vi "play_nPoint_id_slew_OL_FIFO.vi"() -> ()   [LabVIEW 2017]
uses:
  <vilib>/userdefined/High Color/nirio_resource_hc.ctl
  <vilib>/Utility/file.llb/Read Delimited Spreadsheet (DBL).vi
  <vilib>/FPGAPlugInAG/cRIO-9082/niLvFpga_Open_cRIO-9082.vi
  <vilib>/rvi/interface/common/dynamic/niFpgaDynamicAddResources.vi
  <vilib>/FPGAPlugInAG/Dynamic/niLvFpga_Reset_Dynamic.vi
  <vilib>/rvi/interface/common/niFpgaWaitOnOcc.vi
  <vilib>/Utility/error.llb/Error Cluster From Error Code.vi
  <vilib>/rvi/errors/niLvFpgaAdjustHostInterfaceError.vi
  <vilib>/FPGAPlugInAG/Dynamic/niLvFpga_Run_Dynamic.vi
  <vilib>/Utility/file.llb/Write Delimited Spreadsheet (DBL).vi
  <vilib>/FPGAPlugInAG/Dynamic/niLvFpga_Close_Dynamic.vi
  <vilib>/rvi/interface/nirviOpenFPGA/nirviOpenFPGA.xnode
  FPGA Bitfiles/XYpeizocontrol_FPGATargetSPARTA_nPointidslewOLFI_Q7UGYaeAAEs.lvbitx
  <vilib>/rvi/interface/nirviMethod/nirviMethod.xnode
  <vilib>/rvi/interface/nirviReadWriteControl/nirviReadWriteControl.xnode
  <vilib>/rvi/interface/nirviCloseFPGA/nirviCloseFPGA.xnode
  <vilib>/FPGAPlugInAG/Dynamic/niLvFpga_ConfigureFifo_Dynamic.vi
  <vilib>/rvi/errors/niLvFpgaMergeErrorWithErrorCode.vi
  <vilib>/rvi/interface/Simulation/niFpgaSimulationCallBeginRW.vi
  <vilib>/FPGAPlugInAG/Dynamic/niLvFpga_ReadFifo_Dynamic.vi
  NiFpgaLv.dll
  <vilib>/FPGAPlugInAG/Dynamic/niLvFpga_WriteFifo_Dynamic.vi
panel:
  out "elements left":i32=1
  in  "traj_in_path":path
  out "AI1":T1(graph)
  out "size(s) 2":i32[](array[numeric])
  in  "data_out_path":path
  out "AI0":T1(graph)
  out "Waveform Chart":T1(graph)
  out "Loop Done":bool
  in  "Abort":bool
  in  "TsTicks":u32=1600
  out "y iter":i32
  out "size(s)":i32
  in  "umax":dbl=4.0 format="%#_13g"
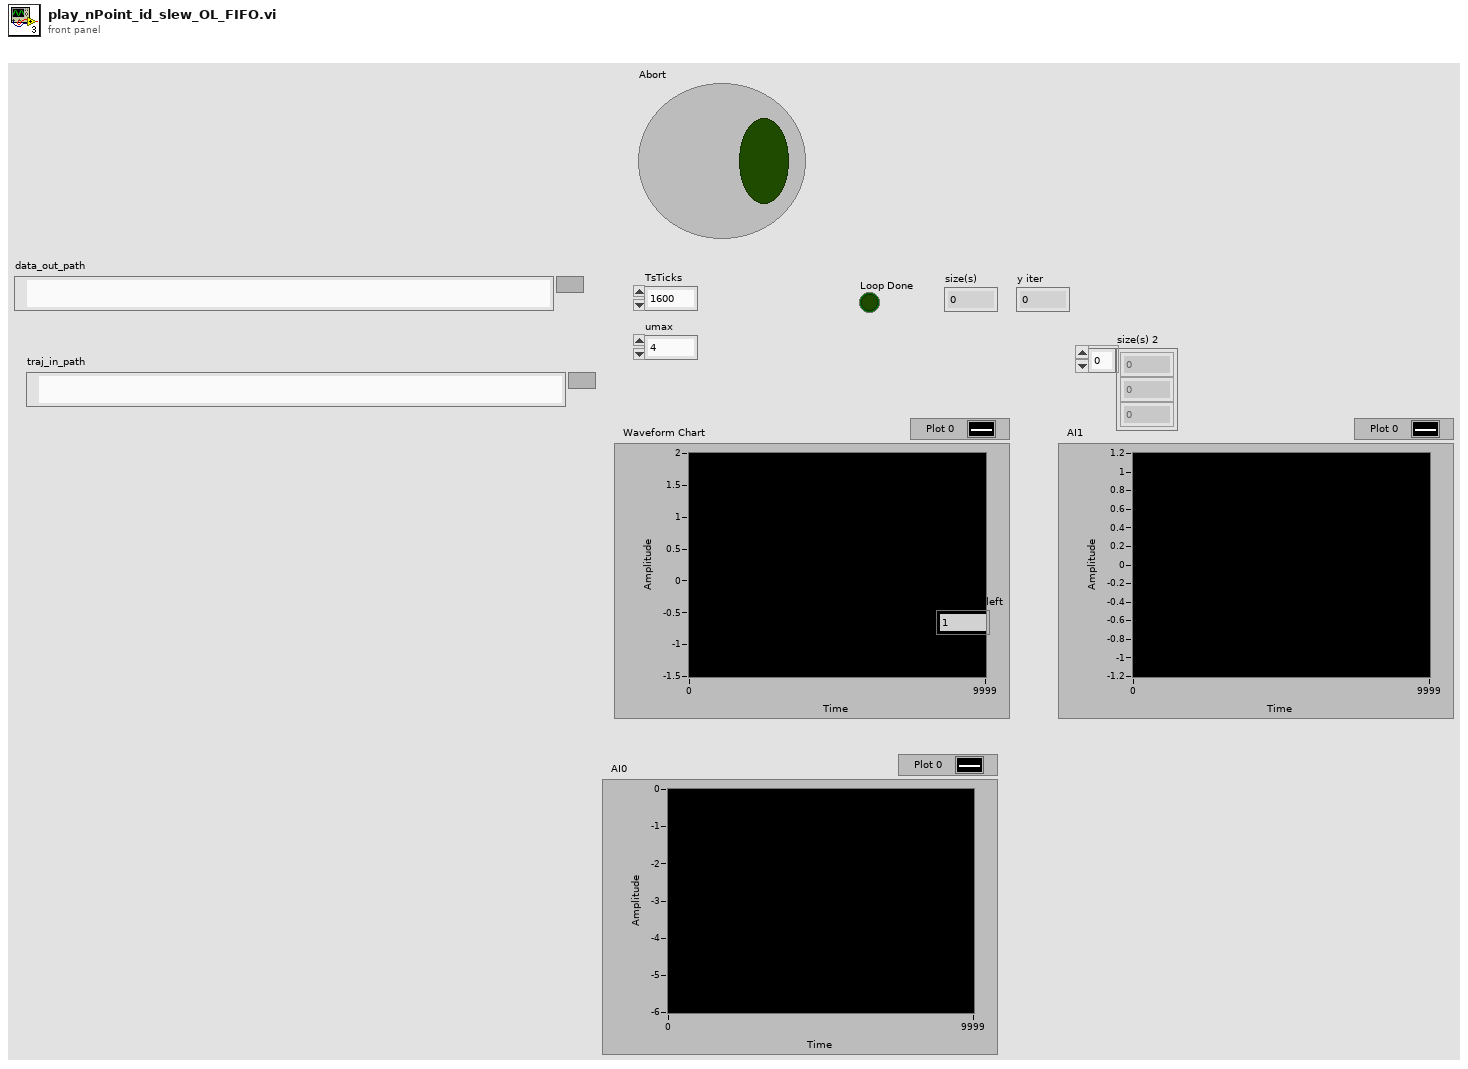
[diagram p1: front panel]
types:
  T1 = cluster{"2D Data Out[0]":dbl, "2D Data Out[1]":dbl, "2D Data Out[2]":dbl, "2D Data Out[3]":dbl, "2D Data Out[4]":dbl, "2D Data Out[5]":dbl, "2D Data Out[6]":dbl, "2D Data Out[7]":dbl, "2D Data Out[8]":dbl}
  T2 = typedef "nirio_resource_hc.ctl" = tag
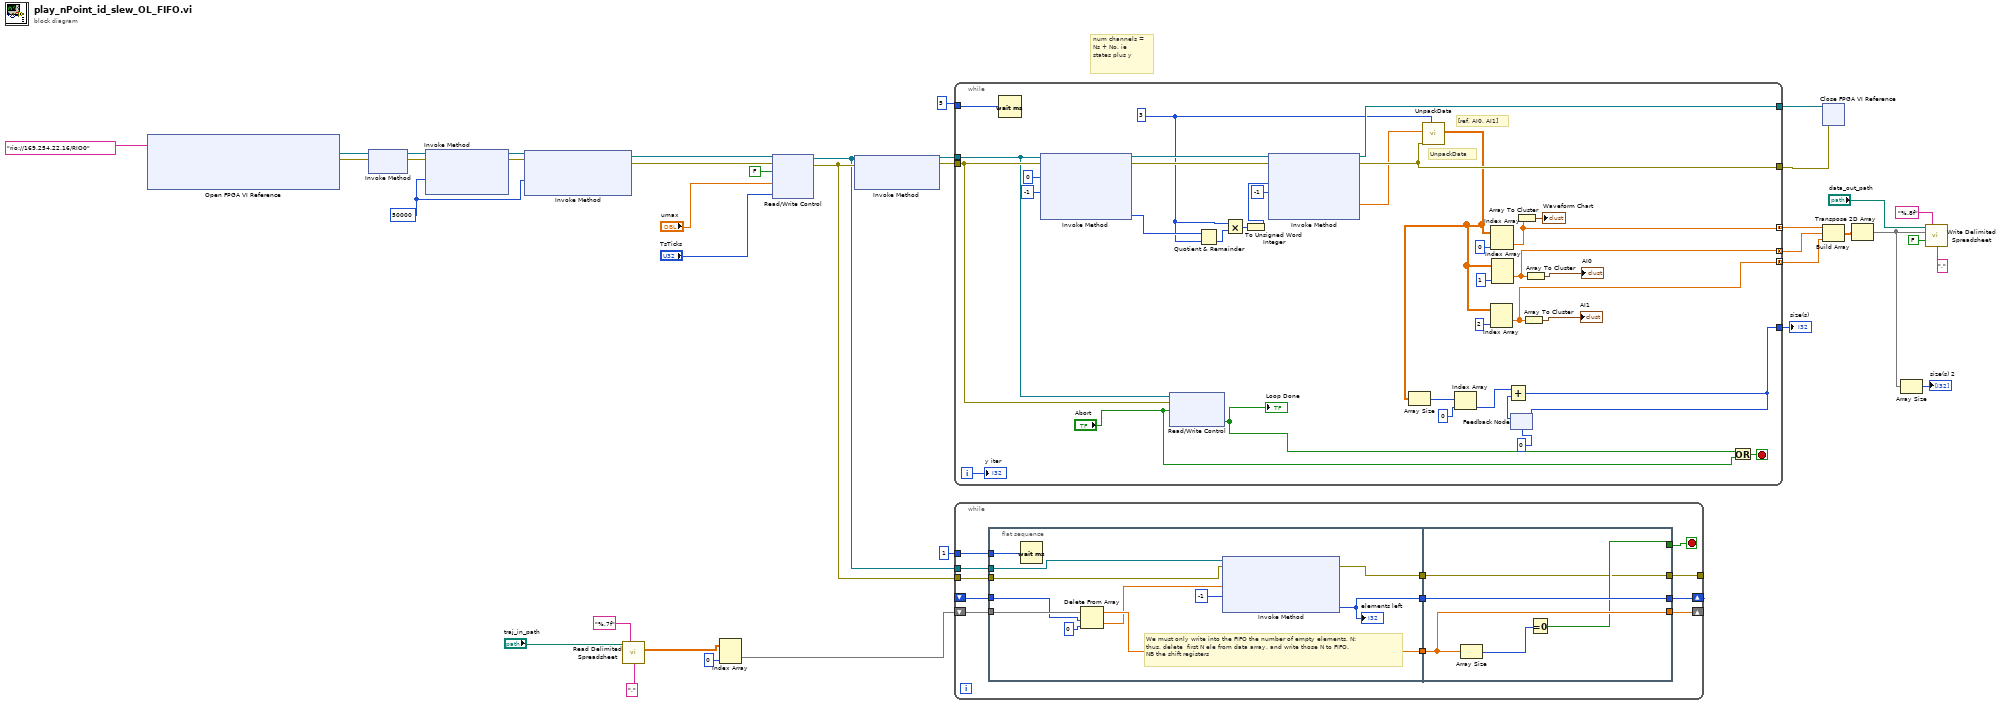
[diagram p0: block diagram]
diagram:
  w7 = 50000
  # "num channels = Ns + No, ie states plus y"
  n1 = xnode "Open FPGA VI Reference"("resource name"=T2 "rio://169.254.22.16/RIO0") -> ("FPGA VI Reference Out"=w34:refnum<k20>, "error out"=w33:errorcluster)  [unwired: 1 in]
  n2 = xnode "Invoke Method"("FPGA VI Reference In"=w34, "error in"=w33) -> ("FPGA VI Reference Out"=w28:refnum<k20>, "error out"=w27:errorcluster)
  n3 = xnode "Invoke Method"("FPGA VI Reference In"=w28, "error in"=w27, "Requested Depth"=w7) -> ("FPGA VI Reference Out"=w11:refnum<k20>, "error out"=w10:errorcluster)  [unwired: 1 out]
  n4 = xnode "Invoke Method"("FPGA VI Reference In"=w11, "error in"=w10, "Requested Depth"=w7) -> ("FPGA VI Reference Out"=w9:refnum<k20>, "error out"=w8:errorcluster)  [unwired: 1 out]
  n5 = call-poly <vilib>:"Read Delimited Spreadsheet.vi"("file path (dialog if empty)"="traj_in_path", "format (%.3f)"="%.7f", "delimiter (\\t)"="," ("delimiter (\\t)")) -> ("all rows"=w3:dbl[][])  [unwired: 7 in, 5 out]
  n6 = Index Array(array=w3, index (col)=0 ("disabled index (col)")) -> (element=w1:dbl[])  [unwired: 1 in]
  n7 = xnode "Read/Write Control"("FPGA VI Reference In"=w9, "error in"=w8, "Abort"=FALSE, "ymax"="umax", "TsTicks"="TsTicks") -> ("FPGA VI Reference Out"=w5:refnum<k20>, "error out"=w6:errorcluster)
  n8 = xnode "Invoke Method"("FPGA VI Reference In"=w5, "error in"=w6) -> ("FPGA VI Reference Out"=w31:refnum<k20>, "error out"=w30:errorcluster)  [unwired: 1 in]
  n9 = while {
    tunnel: 5 -> [w74]
    tunnel: w31 -> [w51]
    tunnel: w30 -> [w52]
    tunnel: [w66] -> w25
    tunnel: [w65] -> w36
    tunnel: [w55] -> w35
    tunnel: [w44] -> w24 mode=concatenating
    tunnel: [w43] -> w23 mode=concatenating
    tunnel: [w39] -> w15 mode=concatenating
    i -> [w56]
    stop <- w54 stop-if-true
    w53 = u32 3 ("y")
    # "[ref, AI0, AI1]"
    # "UnpackData"
    n10 = Wait (ms)(milliseconds to wait=w74) -> ()  [unwired: 1 out]
    n11 = xnode "Invoke Method"("FPGA VI Reference In"=w51, "error in"=w52, "Number of Elements"=0 ("Timeout (ms)"), "Timeout (ms)"=-1) -> ("FPGA VI Reference Out"=w70:refnum<k20>, "error out"=w71:errorcluster, "Elements Remaining"=w62:u32)  [unwired: 1 out]
    n12 = xnode "Read/Write Control"("FPGA VI Reference In"=w51, "error in"=w52, "Abort"="Abort") -> ("Loop Done"=w49:bool)  [unwired: 2 out]
    "Loop Done" <- w49
    n13 = Quotient & Remainder(x=w62, y=w53) -> (floor(x/y)=w63:u32)  [unwired: 1 out]
    n14 = Multiply(x=w53, y=w63) -> (x*y=w68:u32)
    n15 = To Unsigned Word Integer(number=w68) -> (unsigned 16bit integer=w64:u16)
    n16 = xnode "Invoke Method"("FPGA VI Reference In"=w70, "error in"=w71, "Number of Elements"=w64, "Timeout (ms)"=-1) -> ("FPGA VI Reference Out"=w65:refnum<k20>, "error out"=w66:errorcluster, "Data"=w61:sgl[])  [unwired: 1 out]
    n17 = call "UnpackData.vi"("NumChannels"=w53, "error In"=w66, "1D Data In"=w61) -> ("2D Data Out"=w40:dbl[][])  [unwired: 7 in, 1 out]
    n18 = Array Size(array=w40) -> (size(s)=w60:i32[])
    n19 = Index Array(array=w60, index=0) -> (element=w58:i32)
    n20 = Index Array(array=w40, index (col)=2 ("disabled index (col)")) -> (element=w39:dbl[])  [unwired: 1 in]
    n21 = Index Array(array=w40, index (col)=0 ("disabled index (col)")) -> (element=w44:dbl[])  [unwired: 1 in]
    n22 = Index Array(array=w40, index (col)=1 ("disabled index (col)")) -> (element=w43:dbl[])  [unwired: 1 in]
    n23 = feedback #1(0) -> (w59:i32)
    n24 = Add(x=w58, y=w59) -> (x+y=w55:i32)
    n25 = feedback-in #1(w55) -> ()
    n26 = Array To Cluster(array=w44) -> (cluster=→"Waveform Chart":T1)
    n27 = Array To Cluster(array=w39) -> (cluster=→"AI1":T1)
    n28 = Array To Cluster(array=w43) -> (cluster=→"AI0":T1)
    n29 = Or(x=w49, y="Abort") -> (x .or. y?=w54:bool)
    "y iter" <- w56
  }
  "size(s)" <- w35
  n30 = while {
    tunnel: [w84] -> _
    tunnel: 1 -> [w86]
    shift-right: [w79] -> _
    shift-left: _ -> [w83]
    shift-right: [w77] -> _
    shift-left: w1 -> [w85]
    tunnel: w5 -> [w76]
    tunnel: w6 -> [w75]
    stop <- w80 stop-if-true
    n31 = flat-sequence {
      tunnel: w86 -> [w97]
      tunnel: w85 -> [w92]
      tunnel: w83 -> [w88]
      tunnel: [w95] -> w82
      tunnel: [w93] -> w81
      tunnel: [w94] -> w78
      tunnel: w76 -> [w90]
      tunnel: w75 -> [w89]
      tunnel: [w102] -> w79
      tunnel: [w98] -> w84
      tunnel: w82 -> [w98]
      tunnel: w81 -> [w102]
      tunnel: [w99] -> w80
      tunnel: w78 -> [w100]
      tunnel: [w100] -> w77
      frame #0 {
        # "We must only write into the FIFO the number of empty elements, N:\nthus, delete  first N ele from data array, and write those N to FIFO.\nNB the shift registers"
        n32 = Wait (ms)(milliseconds to wait=w97) -> ()  [unwired: 1 out]
        n33 = Delete From Array(array=w92, length=w88, index=0) -> (deleted portion=w91:dbl[], array with subset deleted=w94:dbl[])
        n34 = xnode "Invoke Method"("FPGA VI Reference In"=w90, "error in"=w89, "Data"=w91, "Timeout (ms)"=-1) -> ("error out"=w95:errorcluster, "Empty Elements Remaining"=w93:u32)  [unwired: 1 out]
        "elements left" <- w93
      }
      frame #1 {
        n35 = Array Size(array=w100) -> (size(s)=w101:i32)
        n36 = Equal To 0?(x=w101) -> (x = 0?=w99:bool)
      }
    }
  }
  n37 = xnode "Close FPGA VI Reference"("FPGA VI Reference In"=w36, "error in"=w25) -> ()  [unwired: 1 out]
  n38 = Build Array(w24, w23, w15) -> (w17:dbl[][])
  n39 = Transpose 2D Array(2D array=w17) -> (transposed array=w16:dbl[][])
  n40 = Array Size(array=w16) -> (size(s)=→"size(s) 2":i32[])
  n41 = call-poly <vilib>:"Write Delimited Spreadsheet.vi"("file path (dialog if empty)"="data_out_path", "format (%.3f)"="%.8f", "2D data"=w16, "append to file? (new file:F)"=FALSE, "delimiter (\\t)"="," ("delimiter (\\t)")) -> ()  [unwired: 9 in, 2 out]
